vi "Delete BrowerTree Component.vi"(6 "Delete Children?(True)":bool=TRUE, 8 "error in (no error)":errorcluster, 10 "BrowerComponentID(\"\")":string, 11 "BrowerTree in":refnum<class "BrowerTree.lvclass">) -> (0 "error out":errorcluster, 3 "BrowerTree out":refnum<class "BrowerTree.lvclass">)   [LabVIEW 2015, in "BrowerTree.lvclass"]
uses:
  BrowerTree.lvclass
  BrowerTree.lvclass/BrowerTree.ctl
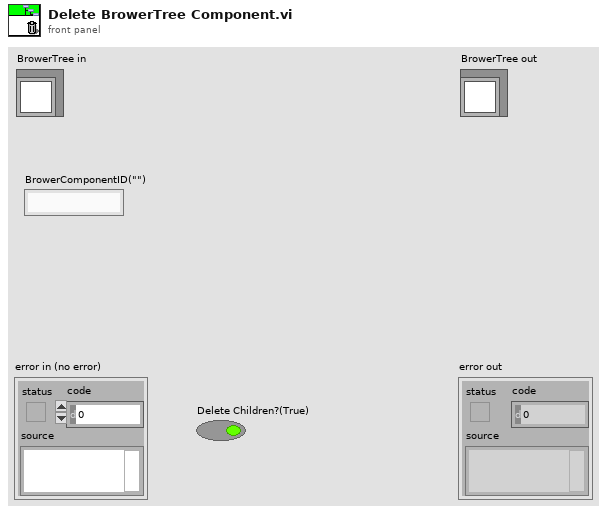
[diagram p1: front panel]
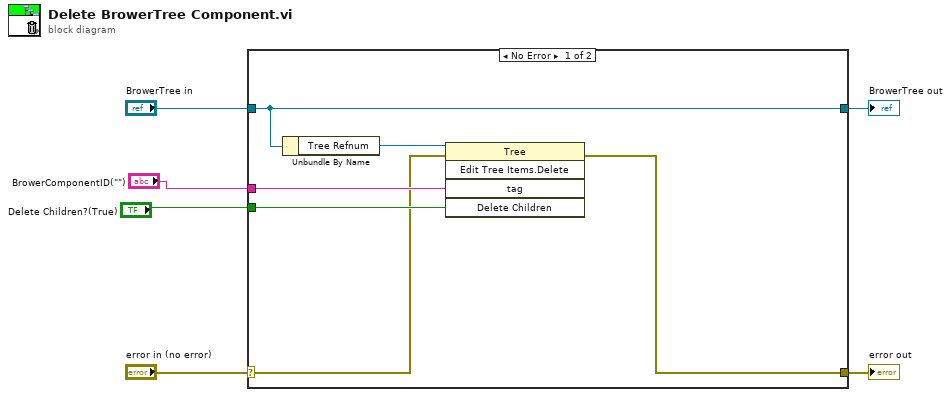
[diagram p0: block diagram]
diagram:
  n1 = case shown="No Error" "error in (no error)" {
    selector: "error in (no error)" -> [w8 w14]
    tunnel: [w7 w14] -> w5
    tunnel: [w12 w13] -> w3
    tunnel: "BrowerTree in" -> [w12 w13]
    tunnel: "BrowerComponentID(\"\")" -> [w10 _]
    tunnel: "Delete Children?(True)" -> [w9 _]
    frame No Error {
      n2 = Unbundle By Name(w12) -> ("Tree Refnum"=w11:refnum<vi>)
      n3 = invoke class="Tree" method="Edit Tree Items.Delete"(reference=w11, error in=w8, "tag"=w10, "Delete Children"=w9) -> (error out=w7:errorcluster)  [unwired: 1 in, 4 out]
    }
    frame Error {
    }
  }
  "error out" <- w5
  "BrowerTree out" <- w3
